vi "WPI_AccumulatorVerifyChannel.vi"(8 "error in (no error)":errorcluster, 11 "AIDeviceRef":T1={"DevStatus"={"status"=FALSE, "code"=0, "source"=""}, "Analog Channel"=enum."AI 1"}) -> (0 "error out":errorcluster, 3 "AIDeviceRef":T1={"DevStatus"={"status"=FALSE, "code"=0, "source"=""}, "Analog Channel"=enum."AI 1"})   [LabVIEW 2017]
doc: "* Initialize the accumulator.\n This is a commmon method for initializing the accumulator for any constructor.\n @param module The analog input module number containing the channel to accumulate.\n @param channel The channel number withing the module that is accumulated.\n @param raw True if the the raw analog values are accumulated, false if the averaged and oversampled values are accumulated.\n \n\n\nThis software is licensed. Open the labview\\readme\\WPI Robotics Library Open Source License.txt file for more information."
uses:
  <vilib>/Rock Robotics/WPI/AnalogChannel/WPI_AnalogChannelDevRef.ctl
  <vilib>/Rock Robotics/SystemInterfaces/AI/FPGA_AIChannel.ctl
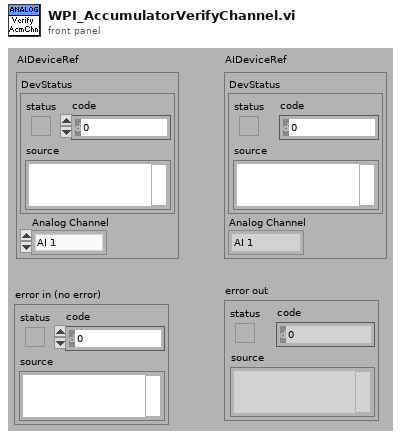
[diagram p1: front panel]
types:
  T1 = typedef "WPI_AnalogChannelDevRef.ctl" = cluster{"DevStatus":errorcluster, "Analog Channel":T2}
  T2 = typedef "FPGA_AIChannel.ctl" = enum8{"AI 0", "AI 1", "AI 2", "AI 3", "AI MXP 0", "AI MXP 1", "AI MXP 2", "AI MXP 3", "Invalid"}
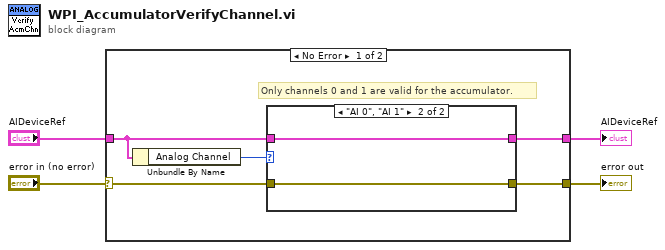
[diagram p0: block diagram]
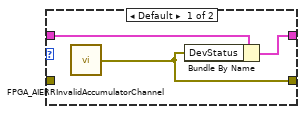
[diagram p2: hidden frame]
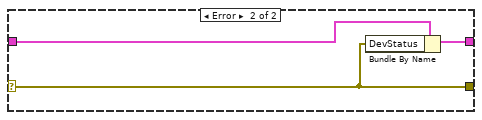
[diagram p3: hidden frame]
diagram:
  n1 = case shown="No Error" "error in (no error)" {
    selector: "error in (no error)" -> [w5 w16]
    tunnel: [w8 w16] -> w4
    tunnel: "AIDeviceRef" -> [w7 w15]
    tunnel: [w6 w17] -> w2
    frame No Error {
      # "Only channels 0 and 1 are valid for the accumulator."
      n2 = Unbundle By Name(w7) -> ("Analog Channel"=w9:T2)
      n3 = case shown="\"AI 0\", \"AI 1\"" w9 {
        tunnel: w5 -> [_ w14]
        tunnel: [w10 w14] -> w8
        tunnel: w7 -> [w12 w13]
        tunnel: [w11 w13] -> w6
        frame Default {
          n4 = call <vilib>:"FPGA_AIERRInvalidAccumulatorChannel.vi"() -> ("error out"=w10:errorcluster)  [unwired: 1 in]
          n5 = Bundle By Name(cluster=w12, "DevStatus"=w10) -> (w11:T1)
        }
        frame "AI 0", "AI 1" {
        }
      }
    }
    frame Error {
      n6 = Bundle By Name(cluster=w15, "DevStatus"=w16) -> (w17:T1)
    }
  }
  "AIDeviceRef" <- w2
  "error out" <- w4
